vi "Perform Step.vi"(8 "error in (no error)":errorcluster, 9 "Keyboard":refnum<k1>, 10 "Hotkeys":T2, 11 "Step":T3={"Type"=enum."Mouse Move", "X"=0, "Y"=0, "Delay"=0, "Key"=65, "Repeat"=0, "RClick?"=FALSE, "App/Window Name"="", "Notes"="", "Assertion Type"=enum."Control Position", "Control Name"="", "Disabled"=enum."Enabled", "Visible"=enum."Visible", "Left"=0, "Top"=0, "Width"=0, "Height"=0, "Expected Image"={"image type"=0, "image depth"=0, "image"=[], "mask"=[], "colors"=[], "Rectangle"={"left"=0, "top"=0, "right"=0, "bottom"=0}}}) -> (0 "error out":errorcluster, 2 "Report Data":T1, 3 "State(s)":string)   [LabVIEW 2020, in "MacroAssert.lvlib"]
doc: "Executes <B>Step</B>, checks for an abort hotkey press, and outputs the next state for the state machine to execute based on the step and <B>Repeat Count</B>."
uses:
  MacroAssert.lvlib
  ec44d10e-72d8-4c7e-b1c7-11b5471dc187.vi
  CTLs/Hotkey Type.ctl
  CTLs/FGV Actions.ctl
  labview_win_util32_8.6/Winevent/Winevent.lvlib
  0fc491d1-540b-4e3c-a9f1-d515ab3959d5.vi
  eed0c13c-4c8d-4811-bf1b-886c68460aaa.vi
  27aa0f71-d9e0-4e00-a40a-04ebf7167400.vi
  70c2b0c9-e855-47dc-a99c-854f52cf3209.vi
  2266d4d6-2cac-4868-b53d-76dc73e57a79.vi
  f6af166c-5c2a-40ab-b52b-e7588615a589.vi
  1d40764d-0ee2-42e1-b1e2-1dce413207b4.vi
  CTLs/Step Type V3.ctl
  labview_win_util32_8.6/Win Util New/Win Util New.lvlib
  CTLs/Report Data.ctl
  CTLs/Hotkey Values.ctl
  CTLs/Step V3.ctl
  CTLs/Assertion Type.ctl
  <vilib>/picture/picture.llb/imagedata.ctl
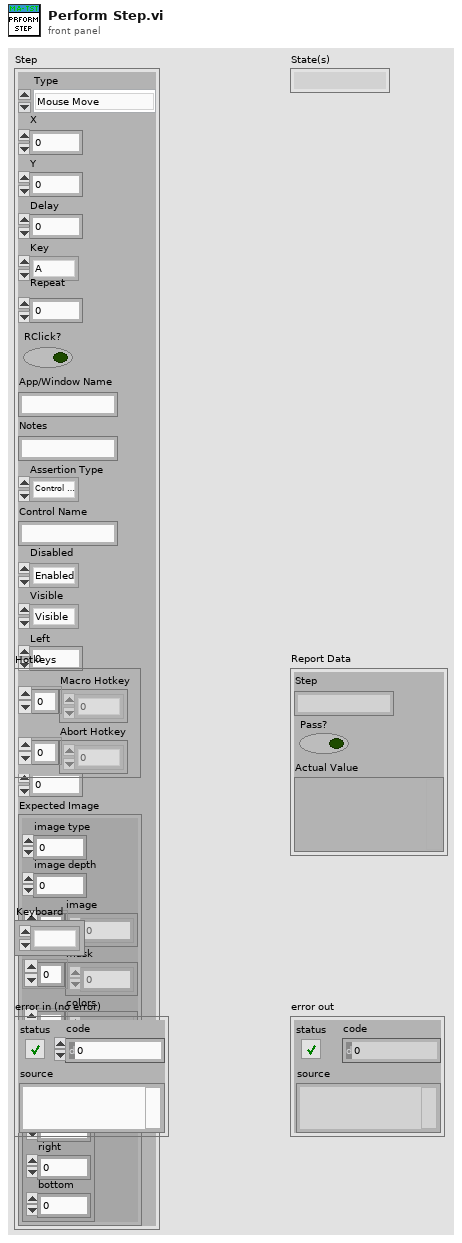
[diagram p1: front panel]
types:
  T1 = typedef "MacroAssert.lvlib/Report Data.ctl" = cluster{"Step":string, "Pass?":bool, "Actual Value":variant}
  T2 = typedef "MacroAssert.lvlib/Hotkey Values.ctl" = cluster{"Macro Hotkey":enum16{"0", "1", "2", "3", "4", "5", "6", "7", "8", "9", "A", "B", "C", "D", "E", "F", "G", "H", "I", "J", "K", "L", "M", "N", "O", "P", "Q", "R", "S", "T", "U", "V", "W", "X", "Y", "Z", "F1", "F2", "F3", "F4", "F5", "F6", "F7", "F8", "F9", "F10", "F11", "F12", "F13", "F14", "F15", "ADD", "BACK", "BACKSLASH", "CAPITAL", "COMMA", "DECIMAL", "DELETE", "DIVIDE", "DOWN", "END", "EQUALS", "ESCAPE", "GRAVE (`)", "HOME", "INSERT", "LBRACKET", "LCONTROL", "LEFT", "L ALT", "LSHIFT", "LWIN", "MINUS", "MULTIPLY", "NEXT", "NUMLOCK", "NUMPAD_0", "NUMPAD_1", "NUMPAD_2", "NUMPAD_3", "NUMPAD_4", "NUMPAD_5", "NUMPAD_6", "NUMPAD_7", "NUMPAD_8", "NUMPAD_9", "PAUSE", "PERIOD", "PRIOR (PG UP)", "RBRACKET", "RCONTROL", "RETURN", "RIGHT", "R ALT", "RSHIFT", "RWIN", "SCROLL", "SEMICOLON", "SLASH", "SPACE", "SUBTRACT", "TAB", "UP", "ENTER (num pad)", "' (quote)"}[], "Abort Hotkey":enum16{"0", "1", "2", "3", "4", "5", "6", "7", "8", "9", "A", "B", "C", "D", "E", "F", "G", "H", "I", "J", "K", "L", "M", "N", "O", "P", "Q", "R", "S", "T", "U", "V", "W", "X", "Y", "Z", "F1", "F2", "F3", "F4", "F5", "F6", "F7", "F8", "F9", "F10", "F11", "F12", "F13", "F14", "F15", "ADD", "BACK", "BACKSLASH", "CAPITAL", "COMMA", "DECIMAL", "DELETE", "DIVIDE", "DOWN", "END", "EQUALS", "ESCAPE", "GRAVE (`)", "HOME", "INSERT", "LBRACKET", "LCONTROL", "LEFT", "L ALT", "LSHIFT", "LWIN", "MINUS", "MULTIPLY", "NEXT", "NUMLOCK", "NUMPAD_0", "NUMPAD_1", "NUMPAD_2", "NUMPAD_3", "NUMPAD_4", "NUMPAD_5", "NUMPAD_6", "NUMPAD_7", "NUMPAD_8", "NUMPAD_9", "PAUSE", "PERIOD", "PRIOR (PG UP)", "RBRACKET", "RCONTROL", "RETURN", "RIGHT", "R ALT", "RSHIFT", "RWIN", "SCROLL", "SEMICOLON", "SLASH", "SPACE", "SUBTRACT", "TAB", "UP", "ENTER (num pad)", "' (quote)"}[]}
  T3 = typedef "MacroAssert.lvlib/Step V3.ctl" = cluster{"Type":T4, "X":i32, "Y":i32, "Delay":i32, "Key":u8, "Repeat":i32, "RClick?":bool, "App/Window Name":string, "Notes":string, "Assertion Type":T5, "Control Name":string, "Disabled":enum8{"Enabled", "Disabled", "Disabled and Grayed Out"}, "Visible":enum16{"Visible", "Not Visible"}, "Left":i16, "Top":i16, "Width":i16, "Height":i16, "Expected Image":T6}
  T4 = typedef "MacroAssert.lvlib/Step Type V3.ctl" = enum16{"Mouse Move", "Mouse Click", "Key Press", "Wait", "Mouse Down", "Mouse Up", "Key Down", "Key Up", "Test Assertion", "Run Application", "Maximize Window", "Restore Window", "Minimize Window", "Close Window", "Bring Window to Front", "Send Window to Back"}
  T5 = typedef "MacroAssert.lvlib/Assertion Type.ctl" = enum16{"Control Position", "Control Visible", "Control Disabled", "Control Image"}
  T6 = typedef "imagedata.ctl" = cluster{"image type":i32, "image depth":i32, "image":u8[], "mask":u8[], "colors":u32[], "Rectangle":cluster{"left":i16, "top":i16, "right":i16, "bottom":i16}}
  T7 = typedef "MacroAssert.lvlib/Hotkey Type.ctl" = enum16{"Macro Hotkey", "Abort Hotkey"}
  T8 = typedef "MacroAssert.lvlib/FGV Actions.ctl" = enum16{"Read", "Write"}
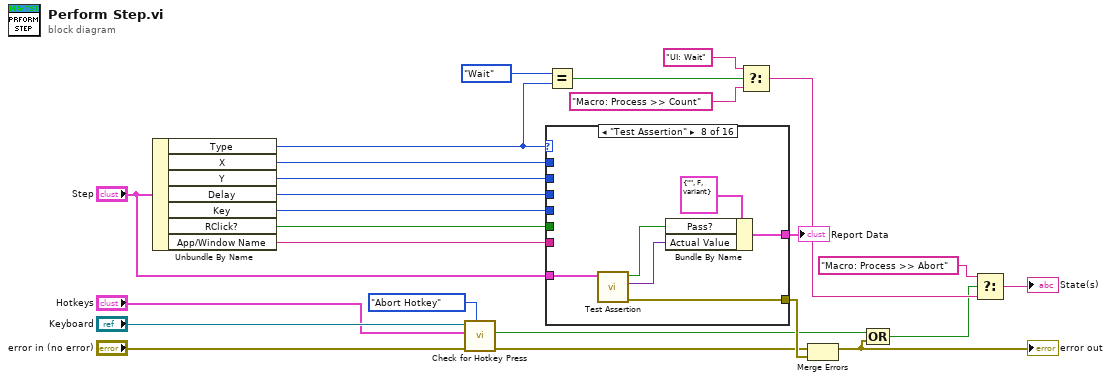
[diagram p0: block diagram]
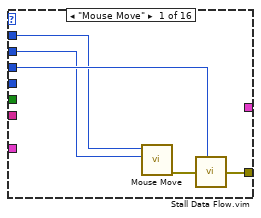
[diagram p2: hidden frame]
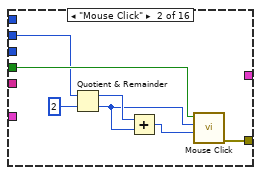
[diagram p3: hidden frame]
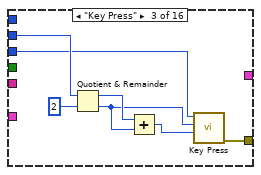
[diagram p4: hidden frame]
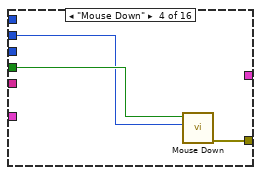
[diagram p5: hidden frame]
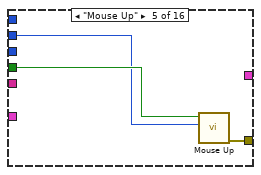
[diagram p6: hidden frame]
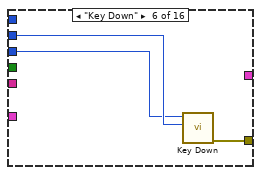
[diagram p7: hidden frame]
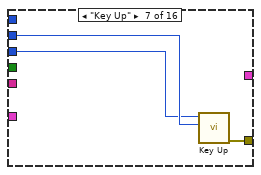
[diagram p8: hidden frame]
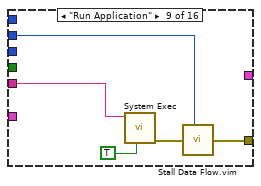
[diagram p9: hidden frame]
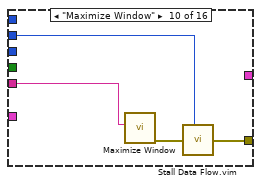
[diagram p10: hidden frame]
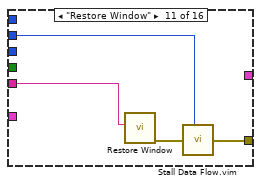
[diagram p11: hidden frame]
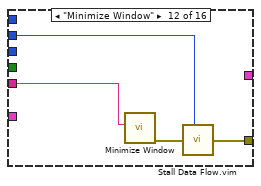
[diagram p12: hidden frame]
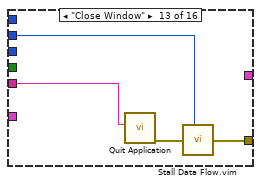
[diagram p13: hidden frame]
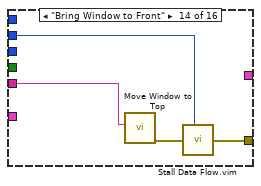
[diagram p14: hidden frame]
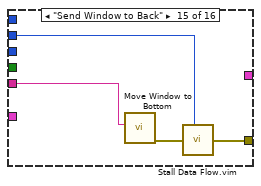
[diagram p15: hidden frame]
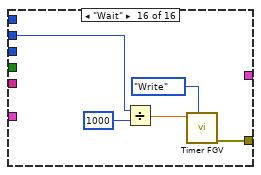
[diagram p16: hidden frame]
diagram:
  n1 = Unbundle By Name("Step") -> ("Type"=w5:T4, "X"=w25:i32, "Y"=w8:i32, "Delay"=w24:i32, "Key"=w23:u8, "RClick?"=w22:bool, "App/Window Name"=w9:string)
  n2 = call "Check for Hotkey Press.vi"("Hotkey Type"=Hotkey_Type."Abort Hotkey", "error in (no error)"="error in (no error)", "Hotkeys"="Hotkeys", "Keyboard"="Keyboard") -> ("error out"=w14:errorcluster, "Pressed?"=w12:bool)  [unwired: 5 in, 1 out]
  n3 = case shown="\"Test Assertion\"" w5 {
    tunnel: w25 -> [w27 _ _ _ _ _ _ _ _ _ _ _ _ _ _ _]
    tunnel: w24 -> [w28 w35 w43 w45 w48 w52 w55 _ w65 w68 w72 w76 w80 w84 w88 w96]
    tunnel: w23 -> [_ _ w38 _ _ w51 w54 _ _ _ _ _ _ _ _ _]
    tunnel: [w29 w37 w44 w47 w50 w53 w56 w62 w66 w69 w73 w77 w81 w85 w89 w93] -> w15
    tunnel: w22 -> [_ w36 _ w46 w49 _ _ _ _ _ _ _ _ _ _ _]
    tunnel: w9 -> [_ _ _ _ _ _ _ _ w64 w70 w74 w78 w82 w86 w90 _]
    tunnel: w8 -> [w26 _ _ _ _ _ _ _ _ _ _ _ _ _ _ _]
    tunnel: [_ _ _ _ _ _ _ w58 _ _ _ _ _ _ _ _] -> w2
    tunnel: "Step" -> [_ _ _ _ _ _ _ w57 _ _ _ _ _ _ _ _]
    frame "Mouse Move" {
      n4 = call "Mouse Move.vi"("y"=w26, "x"=w27) -> ("error out"=w30:errorcluster)  [unwired: 9 in]
      n5 = call "Stall Data Flow.vim"("value in"=w30, "milliseconds to wait"=w28) -> ("value out"=w29:errorcluster)  [unwired: 1 out]
    }
    frame "Mouse Click" {
      n6 = Quotient & Remainder(x=w35, y=2) -> (x-y*floor(x/y)=w33:i32, floor(x/y)=w31:i32)
      n7 = Add(x=w33, y=w31) -> (x+y=w32:i32)
      n8 = call "Mouse Click.vi"("ms wait after up (10)"=w32, "ms wait after down (10)"=w31, "Right Click? (F)"=w36) -> ("error out"=w37:errorcluster)  [unwired: 8 in]
    }
    frame "Key Press" {
      n9 = Quotient & Remainder(x=w43, y=2) -> (x-y*floor(x/y)=w41:i32, floor(x/y)=w39:i32)
      n10 = Add(x=w41, y=w39) -> (x+y=w40:i32)
      n11 = call "Key Press.vi"("ms wait after up (20)"=w40, "ms wait after down (80)"=w39, "Virtual Key"=w38) -> ("error out"=w44:errorcluster)  [unwired: 8 in]
    }
    frame "Mouse Down" {
      n12 = call "Mouse Down.vi"("Delay in ms (10)"=w45, "Right Click? (F)"=w46) -> ("error out"=w47:errorcluster)  [unwired: 9 in]
    }
    frame "Mouse Up" {
      n13 = call "Mouse Up.vi"("Delay in ms (10)"=w48, "Right Click? (F)"=w49) -> ("error out"=w50:errorcluster)  [unwired: 9 in]
    }
    frame "Key Down" {
      n14 = call "Key Down.vi"("delay in ms (80)"=w52, "Virtual Key"=w51) -> ("error out"=w53:errorcluster)  [unwired: 9 in]
    }
    frame "Key Up" {
      n15 = call "Key Up.vi"("delay in ms (20)"=w55, "Virtual Key"=w54) -> ("error out"=w56:errorcluster)  [unwired: 9 in]
    }
    frame "Test Assertion" {
      n16 = call "Test Assertion.vi"("Step"=w57) -> ("error out"=w62:errorcluster, "Actual Value"=w59:variant, "Pass?"=w60:bool)  [unwired: 8 in]
      n17 = Bundle By Name(cluster=T1 {"Step"="", "Pass?"=FALSE, "Actual Value"=variant} ("Report Data"), "Pass?"=w60, "Actual Value"=w59) -> (w58:T1)
    }
    frame "Run Application" {
      n18 = call <vilib>:"System Exec.vi"("run minimized? (F)"=TRUE, "command line"=w64) -> ("error out"=w67:errorcluster)  [unwired: 6 in, 3 out]
      n19 = call "Stall Data Flow.vim"("value in"=w67, "milliseconds to wait"=w65) -> ("value out"=w66:errorcluster)  [unwired: 1 out]
    }
    frame "Maximize Window" {
      n20 = call "Maximize Window.vi"("window name (\"\")"=w70) -> ("error out"=w71:errorcluster)  [unwired: 9 in, 1 out]
      n21 = call "Stall Data Flow.vim"("value in"=w71, "milliseconds to wait"=w68) -> ("value out"=w69:errorcluster)  [unwired: 1 out]
    }
    frame "Restore Window" {
      n22 = call "Restore Window.vi"("window name (\"\")"=w74) -> ("error out"=w75:errorcluster)  [unwired: 9 in, 1 out]
      n23 = call "Stall Data Flow.vim"("value in"=w75, "milliseconds to wait"=w72) -> ("value out"=w73:errorcluster)  [unwired: 1 out]
    }
    frame "Minimize Window" {
      n24 = call "Minimize Window.vi"("window name (\"\")"=w78) -> ("error out"=w79:errorcluster)  [unwired: 9 in, 1 out]
      n25 = call "Stall Data Flow.vim"("value in"=w79, "milliseconds to wait"=w76) -> ("value out"=w77:errorcluster)  [unwired: 1 out]
    }
    frame "Close Window" {
      n26 = call "Quit Application.vi"("window name (\"\")"=w82) -> ("error out"=w83:errorcluster)  [unwired: 10 in]
      n27 = call "Stall Data Flow.vim"("value in"=w83, "milliseconds to wait"=w80) -> ("value out"=w81:errorcluster)  [unwired: 1 out]
    }
    frame "Bring Window to Front" {
      n28 = call "Move Window to Top.vi"("window name (\"\")"=w86) -> ("error out"=w87:errorcluster)  [unwired: 9 in, 1 out]
      n29 = call "Stall Data Flow.vim"("value in"=w87, "milliseconds to wait"=w84) -> ("value out"=w85:errorcluster)  [unwired: 1 out]
    }
    frame "Send Window to Back" {
      n30 = call "Move Window to Bottom.vi"("window name (\"\")"=w90) -> ("error out"=w91:errorcluster)  [unwired: 9 in, 1 out]
      n31 = call "Stall Data Flow.vim"("value in"=w91, "milliseconds to wait"=w88) -> ("value out"=w89:errorcluster)  [unwired: 1 out]
    }
    frame "Wait" {
      n32 = Divide(x=w96, y=1000) -> (x/y=w92:dbl)
      n33 = call "Timer FGV.vi"("Mode"=FGV_Actions."Write", "Timer Value (s)"=w92) -> ("error out"=w93:errorcluster)  [unwired: 7 in, 2 out]
    }
  }
  "Report Data" <- w2
  n34 = Equal?(x=Step_Type_V3."Wait", y=w5) -> (x = y?=w3:bool)
  n35 = Select(t="UI: Wait", s=w3, f="Macro: Process >> Count") -> (s? t:f=w11:string)
  n36 = Merge Errors(w14, w15) -> (w19:errorcluster)
  "error out" <- w19
  n37 = Compound Arithmetic op=OR(w12, w19) -> (w10:bool)
  n38 = Select(t="Macro: Process >> Abort", s=w10, f=w11) -> (s? t:f=→"State(s)":string)
